vi "Read Instances.vi"(8 "error in (no error)":errorcluster, 11 "Lookup Table in":refnum<class "Lookup Table.lvclass">) -> (0 "error out":errorcluster, 2 "Scaling Instances":string[](array[string]), 3 "Lookup Table out":refnum<class "Lookup Table.lvclass">)   [LabVIEW 2024, in "Lookup Table.lvclass"]
doc: "Lookup Table.lvclass:Read Instances.vi\n\nThis VI assembles a list of the names of all the lookup tables defined in the current configuration file.\n\nInstrument Communication Module Version 1.0\nSeptember, 2017 Original Code Consulting David Thomson\n www.originalcode.com"
uses:
  Lookup Table.lvclass
  Lookup Table.lvclass/Lookup Table.ctl
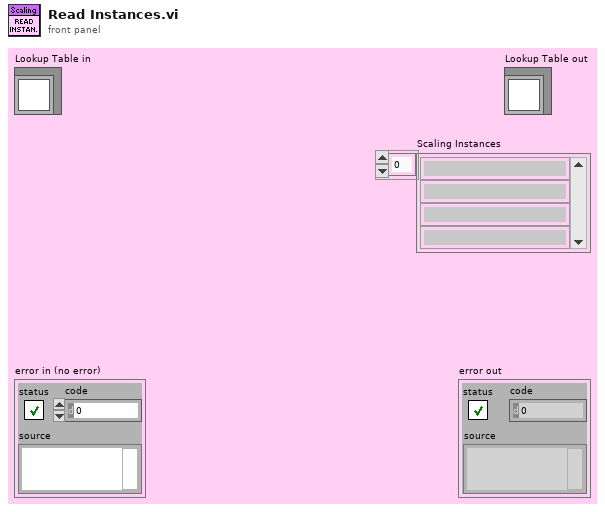
[diagram p1: front panel]
types:
  T1 = cluster{"Instance":string, "Table":cluster{"Raw Value":dbl, "Scaled Value":dbl}[]}[]
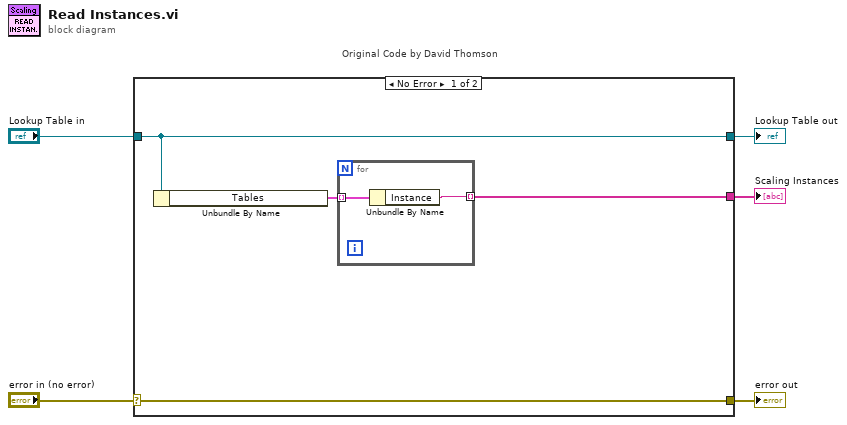
[diagram p0: block diagram]
diagram:
  n1 = case "Original Code by David Thomson" shown="No Error" "error in (no error)" {
    selector: "error in (no error)" -> [w9 w13]
    tunnel: [w9 w13] -> w4
    tunnel: [w8 w12] -> w2
    tunnel: "Lookup Table in" -> [w8 w12]
    tunnel: [w6 _] -> w1
    frame No Error {
      n2 = Unbundle By Name(w8) -> ("Tables"=w7:T1)
      n3 = for {
        tunnel: w7 -> [w11] mode=indexing
        tunnel: [w10] -> w6 mode=indexing
        n4 = Unbundle By Name(w11) -> ("Instance"=w10:string)
      }
    }
    frame Error {
    }
  }
  "error out" <- w4
  "Lookup Table out" <- w2
  "Scaling Instances" <- w1
